vi "Binary Get Metadata.vi"(4 "Binary Data":u8[](array[numeric])) -> (1 "Meta":T1={"# Pages"=0, "ODR"=0, "xlRange"=0, "gyroRange"=0, "id"=0, "Samplig Freq [Hz]"=9.980607627666451, "xlRange in g"=0.0, "gyroRange in dps"=0.0} {"id" format="%02d"; "xlRange" format="%02x"; "ODR" format="%02x"})   [LabVIEW 2019]
uses:
  Controls/gyro_control_measurement_settings.ctl
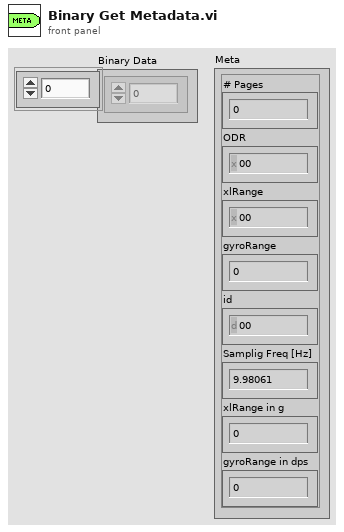
[diagram p1: front panel]
types:
  T1 = typedef "gyro_control_measurement_settings.ctl" = cluster{"# Pages":i32, "ODR":u8, "xlRange":u8, "gyroRange":u8, "id":u8, "Samplig Freq [Hz]":dbl, "xlRange in g":dbl, "gyroRange in dps":dbl}
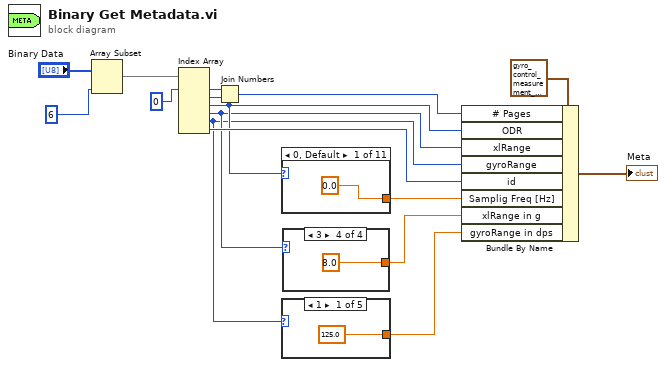
[diagram p0: block diagram]
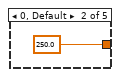
[diagram p2: hidden frame]
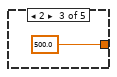
[diagram p3: hidden frame]
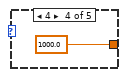
[diagram p4: hidden frame]
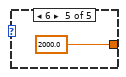
[diagram p5: hidden frame]
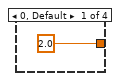
[diagram p6: hidden frame]
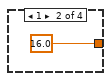
[diagram p7: hidden frame]
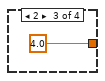
[diagram p8: hidden frame]
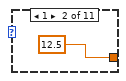
[diagram p9: hidden frame]
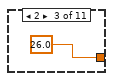
[diagram p10: hidden frame]
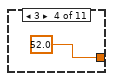
[diagram p11: hidden frame]
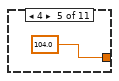
[diagram p12: hidden frame]
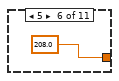
[diagram p13: hidden frame]
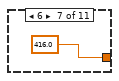
[diagram p14: hidden frame]
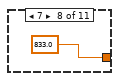
[diagram p15: hidden frame]
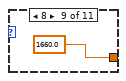
[diagram p16: hidden frame]
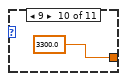
[diagram p17: hidden frame]
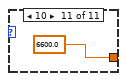
[diagram p18: hidden frame]
diagram:
  n1 = Array Subset(array="Binary Data", length=6 ("index")) -> (w11:u8[])  [unwired: 1 in]
  n2 = Index Array(array=w11, index #1=0 ("index")) -> (element #1=w14:u8, element #2=w13:u8, element #3=w6:u8, element #4=w4:u8, element #5=w2:u8, element #6=w7:u8)  [unwired: 5 in]
  n3 = Join Numbers(hi=w14, lo=w13) -> ((hi.lo)=w8:u16)
  n4 = case shown="0, Default" w6 {
    tunnel: [0.0 ("sampling frequency [Hz]") 12.5 ("sampling frequency [Hz]") 26.0 ("sampling frequency [Hz]") 52.0 ("sampling frequency [Hz]") 104.0 ("sampling frequency [Hz]") 208.0 ("sampling frequency [Hz]") 416.0 ("sampling frequency [Hz]") 833.0 ("sampling frequency [Hz]") 1660.0 ("sampling frequency [Hz]") 3300.0 ("sampling frequency [Hz]") 6600.0 ("sampling frequency [Hz]")] -> w5
    frame 0, Default {
    }
    frame 1 {
    }
    frame 2 {
    }
    frame 3 {
    }
    frame 4 {
    }
    frame 5 {
    }
    frame 6 {
    }
    frame 7 {
    }
    frame 8 {
    }
    frame 9 {
    }
    frame 10 {
    }
  }
  n5 = case shown="1" w2 {
    tunnel: [125.0 ("sampling frequency [Hz]") 250.0 ("sampling frequency [Hz]") 500.0 ("sampling frequency [Hz]") 1000.0 ("sampling frequency [Hz]") 2000.0 ("sampling frequency [Hz]")] -> w1
    frame 1 {
    }
    frame 0, Default {
    }
    frame 2 {
    }
    frame 4 {
    }
    frame 6 {
    }
  }
  n6 = case shown="3" w4 {
    tunnel: [2.0 ("sampling frequency [Hz]") 16.0 ("sampling frequency [Hz]") 4.0 ("sampling frequency [Hz]") 8.0 ("sampling frequency [Hz]")] -> w3
    frame 0, Default {
    }
    frame 1 {
    }
    frame 2 {
    }
    frame 3 {
    }
  }
  n7 = Bundle By Name(cluster=T1 {"# Pages"=0, "ODR"=0, "xlRange"=0, "gyroRange"=0, "id"=0, "Samplig Freq [Hz]"=9.980607627666451, "xlRange in g"=0.0, "gyroRange in dps"=0.0} ("measurement settings"), "# Pages"=w8, "ODR"=w6, "xlRange"=w4, "gyroRange"=w2, "id"=w7, "Samplig Freq [Hz]"=w5, "xlRange in g"=w3, "gyroRange in dps"=w1) -> (→"Meta":T1)
